vi "Create IIR Filter from Cascaded Coefficients.vi"() -> ()   [LabVIEW 2023]
doc: "Demonstrates how to use the DFD Build Filter from Cascaded Coef VI to create a filter from the IIR Filter Cluster generated by the Advanced IIR Filtering VIs in LabVIEW.\n\nComplete the following steps to use this VI.\n1) Run the VI.\n2) Change the specifications.\n3) Observe the IIR Filter Cluster.\n4) Observe the Magnitude Response and Phase Response graphs plotted by the DFD Plot Freq Response VI.\n5) Click the <B>STOP</B> button to stop this VI.\n5) Examine the block diagram of the VI to learn how to use the DFD Build Filter from Cascaded Coef VI to create a filter from the IIR Filter Cluster generated by the Advanced IIR Filtering VIs in LabVIEW."
uses:
  <vilib>/addons/Digital Filter Design/_Objects.llb/DFD Phase Setting.ctl
  <vilib>/addons/Digital Filter Design/Analysis.llb/DFD Plot Freq Response (Linear-Spaced).vi
  <vilib>/Analysis/NI_AALBase.lvlib
  <vilib>/addons/Digital Filter Design/NI_DigFilterLicensed.lvlib
panel:
  out "IIR Filter Cluster":T1 {"Forward Coefficients" format="%.4f"; "Reverse Coefficients" format="%.4f"}
  in  "stop":bool
  out "Error Message":string
  out "Phase Response":cluster{"f0":dbl, "df":dbl, "values":dbl[]}[](graph)
  out "Magnitude Response":cluster{"f0":dbl, "df":dbl, "values":dbl[]}[](graph)
  in  "Order":i32=2
  in  "Low Cutoff Frequency [Hz]":dbl=0.125 format="%0.3f"
  in  "Filter Type":T2(ring)
  in  "High Cutoff Frequency [Hz]":dbl=0.45 format="%0.3f"
  in  "Sampling Frequency [Hz]":dbl=1.0 format="%0.2f"
  in  "Design Method":T3(ring)
  # "Select Help>>Show Context Help and move the cursor over the VI icon for more information."
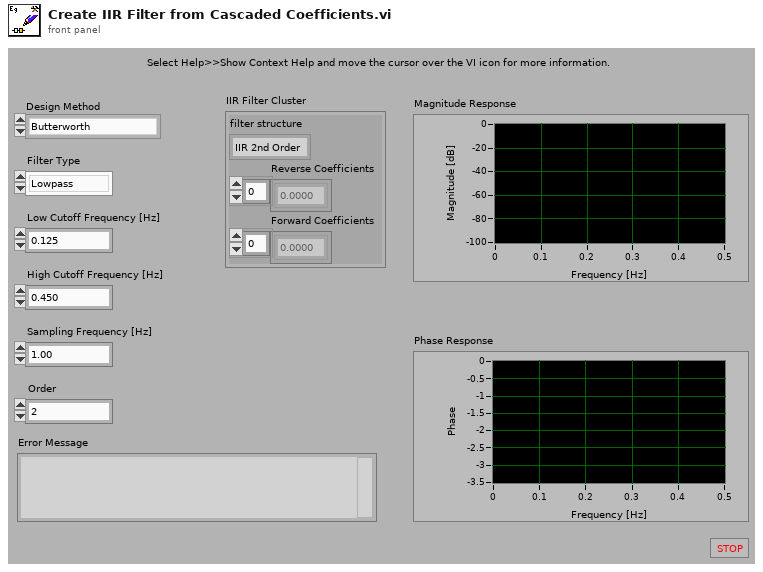
[diagram p1: front panel]
types:
  T1 = cluster{"filter structure":enum32{"IIR 2nd Order", "IIR 4th Order"}, "Reverse Coefficients":dbl[], "Forward Coefficients":dbl[]}
  T2 = enum32{"Lowpass", "Highpass", "Bandpass", "Bandstop"}
  T3 = enum16{"Butterworth", "Chebyshev", "Inv Chebyshev", "Elliptic", "Bessel"}
  T4 = typedef "NI_DigFilterLicensed.lvlib/DFD Phase Setting.ctl" = cluster{"unwrap? (F)":bool, "degree? (F)":bool}
  T5 = typedef "NI_DigFilterLicensed.lvlib/DFD Filter Obj.ctl" = cluster{"mSRate_Fs":dbl, "mSRate_Version":string, "mSRate_Comments":string, "mSRate_OrgCoef":T6, "mSRate_CurCoef":T6, "mSRate_Quantized?":bool, "mSRate_QCoef":T6, "mSRate_QSettings":T8[], "mSRate_Order":i32, "mSRate_Scaling":cluster{"mSRate_ScaleByPowerOf2?":bool, "mSRate_ScaleType":T10}}
  T6 = typedef "NI_DigFilterLicensed.lvlib/DFD Filter Coef.ctl" = cluster{"type":T7, "gain":dbl, "coef a (k)":dbl[], "coef b (v)":dbl[]}
  T7 = typedef "NI_DigFilterLicensed.lvlib/DFD Filter Structure Type Selector.ctl" = enum16{"Undefined", "FIR Direct Form", "FIR Direct Form Transposed", "FIR Symmetric", "FIR Antisymmetric", "IIR Direct Form I", "IIR Direct Form I Transposed", "IIR Direct Form II", "IIR Direct Form II Transposed", "IIR Cascaded Second Order Sections Form I", "IIR Cascaded Second Order Sections Form I Transposed", "IIR Cascaded Second Order Sections Form II", "IIR Cascaded Second Order Sections Form II Transposed", "Lattice Allpass (basic sections)", "Lattice Allpass (one multiplier sections)", "Lattice Allpass (normalized sections)", "Lattice AR (basic sections)", "Lattice AR (one multiplier sections)", "Lattice AR (normalized sections)", "Lattice MA (minimum phase)", "Lattice MA (maximum phase)", "Lattice ARMA (basic sections)", "Lattice ARMA (one multiplier sections)", "Lattice ARMA (normalized sections)"}
  T8 = typedef "NI_DigFilterLicensed.lvlib/dfd_Internal Quantization Settings.ctl" = cluster{"source":T9, "wl":i16, "iwl":i16, "overflow mode":enum16{"Saturation", "Wrap"}, "rounding mode":enum16{"Nearest", "Truncation"}, "signed?":bool}
  T9 = typedef "NI_DigFilterLicensed.lvlib/dfd_Internal Quantization Srcs.ctl" = u16
  T10 = typedef "NI_DigFilterLicensed.lvlib/DFD Coef Norm Type.ctl" = enum16{"No Norm", "Time Domain 1-Norm", "Time Domain 2-Norm", "Time Domain Inf-Norm"}
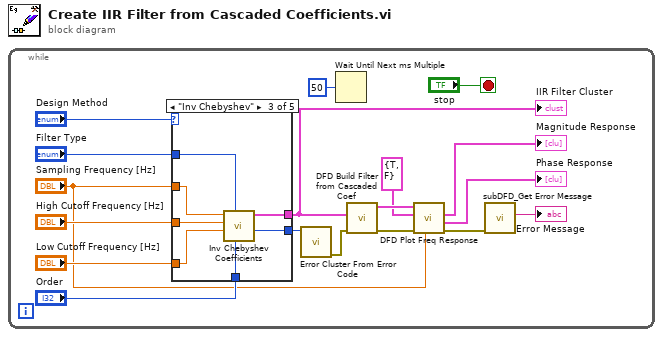
[diagram p0: block diagram]
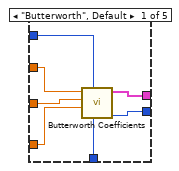
[diagram p2: hidden frame]
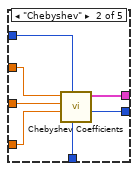
[diagram p3: hidden frame]
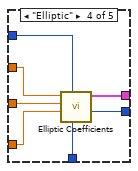
[diagram p4: hidden frame]
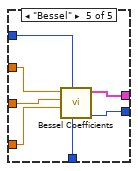
[diagram p5: hidden frame]
diagram:
  n1 = while {
    stop <- "stop" stop-if-true
    n2 = case shown="\"Inv Chebyshev\"" "Design Method" {
      tunnel: "Filter Type" -> [w25 w28 w35 w42 w50]
      tunnel: "Sampling Frequency [Hz]" -> [w24 w32 w38 w45 w53]
      tunnel: "High Cutoff Frequency [Hz]" -> [w23 w31 w39 w46 w52]
      tunnel: "Low Cutoff Frequency [Hz]" -> [w22 w30 w37 w44 w51]
      tunnel: "Order" -> [w21 w29 w36 w43 w49]
      tunnel: [w20 w26 w34 w40 w48] -> w16
      tunnel: [w19 w27 w33 w41 w47] -> w15
      frame "Butterworth", Default {
        n3 = call <vilib>:"Butterworth Coefficients.vi"("order"=w21, "filter type"=w25, "low cutoff freq: fl"=w22, "high cutoff freq: fh"=w23, "sampling freq: fs"=w24) -> ("error"=w20:i32, "IIR Filter Cluster"=w19:T1)  [unwired: 5 in]
      }
      frame "Chebyshev" {
        n4 = call <vilib>:"Chebyshev Coefficients.vi"("order"=w29, "filter type"=w28, "low cutoff freq: fl"=w30, "high cutoff freq: fh"=w31, "sampling freq: fs"=w32) -> ("error"=w26:i32, "IIR Filter Cluster"=w27:T1)  [unwired: 5 in]
      }
      frame "Inv Chebyshev" {
        n5 = call <vilib>:"Inv Chebyshev Coefficients.vi"("order"=w36, "filter type"=w35, "low cutoff freq: fl"=w37, "high cutoff freq: fh"=w39, "sampling freq: fs"=w38) -> ("error"=w34:i32, "IIR Filter Cluster"=w33:T1)  [unwired: 5 in]
      }
      frame "Elliptic" {
        n6 = call <vilib>:"Elliptic Coefficients.vi"("order"=w43, "filter type"=w42, "low cutoff freq: fl"=w44, "high cutoff freq: fh"=w46, "sampling freq: fs"=w45) -> ("error"=w40:i32, "IIR Filter Cluster"=w41:T1)  [unwired: 5 in]
      }
      frame "Bessel" {
        n7 = call <vilib>:"Bessel Coefficients.vi"("order"=w49, "filter type"=w50, "low cutoff freq: fl"=w51, "high cutoff freq: fh"=w52, "sampling freq: fs"=w53) -> ("error"=w48:i32, "IIR Filter Cluster"=w47:T1)  [unwired: 5 in]
      }
    }
    "IIR Filter Cluster" <- w15
    n8 = call <vilib>:"Error Cluster From Error Code.vi"("error code (0)"=w16) -> ("error out"=w14:errorcluster)  [unwired: 2 in, 6 out]
    n9 = Wait Until Next ms Multiple(millisecond multiple=u32 50) -> ()  [unwired: 1 out]
    n10 = call <vilib>:"DFD Build Filter from Cascaded Coef.vi"("error in (no error)"=w14, "IIR Filter Cluster"=w15) -> ("error out"=w12:errorcluster, "filter out"=w13:T5)  [unwired: 1 in, 7 out]
    n11 = call-poly <vilib>:"DFD Plot Freq Response.vi"("fs [Hz]"="Sampling Frequency [Hz]", "error in (no error)"=w12, "phase view"=T4 {"unwrap? (F)"=TRUE, "degree? (F)"=FALSE}, "filter in"=w13) -> ("error out"=w7:errorcluster, "phase response"=→"Phase Response":cluster{"f0":dbl, "df":dbl, "values":dbl[]}[], "magnitude response"=→"Magnitude Response":cluster{"f0":dbl, "df":dbl, "values":dbl[]}[])  [unwired: 4 in, 1 out]
    n12 = call <vilib>:"subDFD_Get Error Message.vi"("error in (no error)"=w7) -> ("Error Message"=→"Error Message":string)  [unwired: 10 out]
  }
